vi "Untitled 2.vi"   [LabVIEW 2020]
uses:
  Data.PG.lvclass
types:
  T1 = cluster{"doubles":dbl[], "integers":i32[], "booleans":bool[], "strings":string[]}
  T2 = cluster{"doubles paths":string[], "integer paths":string[], "boolean paths":string[], "string paths":string[]}
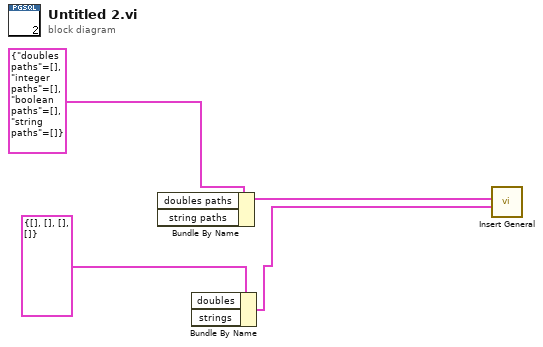
[diagram p0: block diagram]
diagram:
  n1 = Bundle By Name(cluster=T2 {"doubles paths"=[], "integer paths"=[], "boolean paths"=[], "string paths"=[]} ("Paths")) -> (w4:T2)  [unwired: 2 in]
  n2 = Bundle By Name(cluster=T1 {"doubles"=[], "integers"=[], "booleans"=[], "strings"=[]} ("Data")) -> (w1:T1)  [unwired: 2 in]
  n3 = call "Insert General.vi"("Data"=w1, "Paths"=w4) -> ()  [unwired: 8 in, 2 out]
